vi "IR_global.vi"() -> ()   [LabVIEW 2017]
panel:
  in  "IR Range (Right)":dbl
  in  "IR Range (Left)":dbl
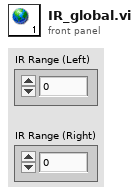
[diagram p1: front panel]
diagram:
